vi "Integer Definition.vi"(11 "Integer in":refnum<class "Integer.lvclass">) -> (2 "Definition":T1)   [LabVIEW 2020, in "Conditum.lvlib" / "Columns.lvlib" / "Integer.lvclass"]
uses:
  Integer.lvclass
  Integer.lvclass/Integer.ctl
  Definition.ctl
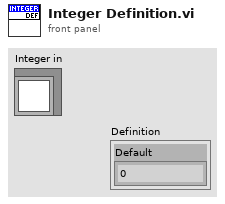
[diagram p1: front panel]
types:
  T1 = typedef "Conditum.lvlib/Columns.lvlib/Integer.lvclass/Definition.ctl" = cluster{"Default":i64}
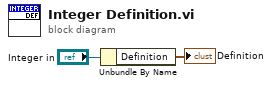
[diagram p0: block diagram]
diagram:
  n1 = Unbundle By Name("Integer in") -> ("Definition"=→"Definition":T1)
